vi "Cannon camera offset.vi"(2 "Compliting angle to 180":dbl, 3 "Distance (from camera)":dbl, 4 "Offset (from center axis to camera lens)":dbl, 5 "Camera angle":dbl) -> (0 "Angle (from cannon to target)":dbl, 1 "Distance from cannon":dbl)   [LabVIEW 2012]
panel:
  # "the left over from the back of the camera"
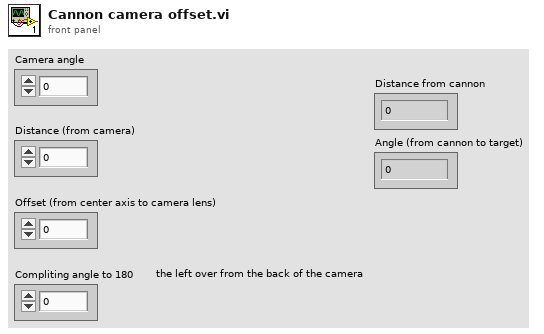
[diagram p1: front panel]
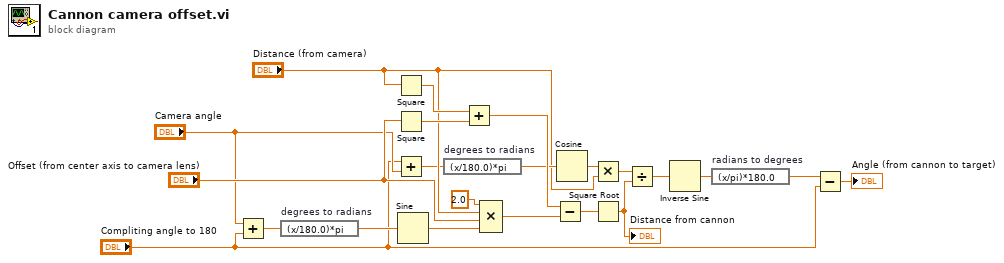
[diagram p0: block diagram]
diagram:
  n1 = Add(x="Camera angle", y="Compliting angle to 180") -> (x+y=w15:dbl)
  n2 = expression code="(x/180.0)*pi" "degrees to radians"(w15) -> (w16:dbl)
  n3 = Square(x="Distance (from camera)") -> (x^2=w18:dbl)
  n4 = Square(x="Offset (from center axis to camera lens)") -> (x^2=w22:dbl)
  n5 = Add(x="Compliting angle to 180", y="Camera angle") -> (x+y=w5:dbl)
  n6 = Sine(x=w16) -> (sin(x)=w13:dbl)
  n7 = expression code="(x/180.0)*pi" "degrees to radians"(w5) -> (w10:dbl)
  n8 = Add(x=w18, y=w22) -> (x+y=w21:dbl)
  n9 = Compound Arithmetic op=MULTIPLY(2.0 ("value"), "Distance (from camera)", "Offset (from center axis to camera lens)", w13) -> (w20:dbl)
  n10 = Subtract(x=w21, y=w20) -> (x-y=w14:dbl)
  n11 = Cosine(x=w10) -> (cos(x)=w9:dbl)
  n12 = Multiply(x=w9, y="Distance (from camera)") -> (x*y=w11:dbl)
  n13 = Square Root(x=w14) -> (sqrt(x)=w7:dbl)
  "Distance from cannon" <- w7
  n14 = Divide(x=w11, y=w7) -> (x/y=w4:dbl)
  n15 = Inverse Sine(1:w4) -> (0:w3:dbl)
  n16 = expression code="(x/pi)*180.0" "radians to degrees"(w3) -> (w2:dbl)
  n17 = Subtract(x=w2, y="Compliting angle to 180") -> (x-y=→"Angle (from cannon to target)":dbl)
